vi "Begin.vi"(8 "error in":errorcluster) -> (0 "error out":errorcluster)   [LabVIEW 2020]
doc: "Called before other user functions, this VI is expected to open initial I/O refnums, load in file data, and do all program initialization. Notice that the <B>error out</B> terminal is simply used for data flow. Wiring it to other structures or subVIs ensures that this VI runs first."
uses:
  <vilib>/Rock Robotics/WPI/Compressor/WPI_CompressorFeedbackMode.ctl
  <vilib>/Rock Robotics/WPI/DriverStation/WPI_DriverStationRobotMode2.ctl
  <vilib>/Rock Robotics/WPI/Joystick/WPI_JoystickDeviceEnum.ctl
  <vilib>/Rock Robotics/WPI/ThirdParty/REV Robotics/REVLib/Typedef/Spark MAX Control Type.ctl
  <vilib>/Rock Robotics/WPI/ThirdParty/Sensors/navX/_TypeDefs/FRIC_navX_DeviceNumbersTypeDef.ctl
  <vilib>/Rock Robotics/WPI/Solenoid/WPI_SolenoidChannel.ctl
  <vilib>/Rock Robotics/SystemInterfaces/DIO/FPGA_DIOPWMChannel.ctl
  <vilib>/Rock Robotics/SystemInterfaces/DIO/FPGA_DIOChannel.ctl
  Robot Global Data.vi
  <vilib>/Rock Robotics/Network Tables/NT Write String Array.vi
  <vilib>/Rock Robotics/WPI/Solenoid/WPI_SolenoidOpenDouble.vi
  <vilib>/Rock Robotics/WPI/Utilities/WPI_GetSetVariantRefNum.vi
  <vilib>/Rock Robotics/WPI/MotorControl/WPI_MotorControlOpen SPARK.vi
  <vilib>/Rock Robotics/WPI/Switch/WPI_SwitchOpenLimit.vi
panel:
  in  "Feedback Configuration":T2={"Feedback Sensor"=enum."Analog Only", "Max Pressure (PSI)"=120.0, "Min Pressure (PSI)"=90.0}
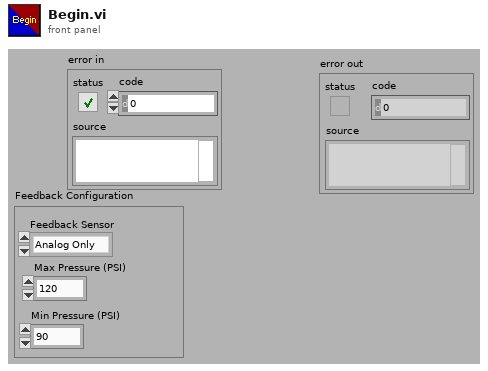
[diagram p1: front panel]
types:
  T1 = typedef "WPI_CompressorFeedbackMode.ctl" = enum16{"Analog Only", "Digital Only", "Hybrid"}
  T2 = cluster{"Feedback Sensor":T1, "Max Pressure (PSI)":dbl, "Min Pressure (PSI)":dbl}
  T3 = typedef "FPGA_DIOChannel.ctl" = enum8{"DIO 0", "DIO 1", "DIO 2", "DIO 3", "DIO 4", "DIO 5", "DIO 6", "DIO 7", "DIO 8", "DIO 9", "DIO MXP 0", "DIO MXP 1", "DIO MXP 2", "DIO MXP 3", "DIO MXP 4", "DIO MXP 5", "DIO MXP 6", "DIO MXP 7", "DIO MXP 8", "DIO MXP 9", "DIO MXP 10", "DIO MXP 11", "DIO MXP 12", "DIO MXP 13", "DIO MXP 14", "DIO MXP 15", "SPI Port CS1", "SPI Port CS2", "SPI Port CS3", "SPI Port MISO", "SPI Port MOSI", "Invalid"}
  T4 = typedef "FPGA_DIOPWMChannel.ctl" = enum8{"PWM 0", "PWM 1", "PWM 2", "PWM 3", "PWM 4", "PWM 5", "PWM 6", "PWM 7", "PWM 8", "PWM 9", "PWM MXP 0", "PWM MXP 1", "PWM MXP 2", "PWM MXP 3", "PWM MXP 4", "PWM MXP 5", "PWM MXP 6", "PWM MXP 7", "PWM MXP 8", "PWM MXP 9", "Invalid"}
  T5 = typedef "WPI_JoystickDeviceEnum.ctl" = enum16{"USB 0", "USB 1", "USB 2", "USB 3", "USB 4", "USB 5"}
  T6 = typedef "WPI_SolenoidChannel.ctl" = enum8{"Solenoid 0", "Solenoid 1", "Solenoid 2", "Solenoid 3", "Solenoid 4", "Solenoid 5", "Solenoid 6", "Solenoid 7", "Solenoid 8", "Solenoid 9", "Solenoid 10", "Solenoid 11", "Solenoid 12", "Solenoid 13", "Solenoid 14", "Solenoid 15", "Invalid"}
  T7 = typedef "Spark MAX Control Type.ctl" = enum16{"Percent VBus", "Voltage", "Velocity", "Position", "Smart Motion", "Current", "Smart Velocity"}
  T8 = typedef "FRIC_navX_DeviceNumbersTypeDef.ctl" = enum16{"Dev0", "Dev1", "Dev2", "Dev3"}
  T9 = typedef "WPI_DriverStationRobotMode2.ctl" = enum16{"Autonomous Disabled", "Autonomous Enabled", "Teleop Disabled", "Teleop Enabled", "Disconnected", "Finish", "Test Disabled", "Test Enabled", "Emergency Stopped"}
  T10 = typedef "WPI_SwitchDevRef.ctl" = cluster{"DevStatus":errorcluster, "DIO Channel":T3, "CntIndex":T11, "Normally Closed":bool}
  T11 = typedef "FPGA_CounterCtrSystemIndex.ctl" = enum8{"Ctr 0", "Ctr 1", "Ctr 2", "Ctr 3", "Ctr 4", "Ctr 5", "Ctr 6", "Ctr 7", "Invalid"}
  T12 = typedef "WPI_SolenoidDevRef.ctl" = cluster{"DevStatus":errorcluster, "Pneumatics Control Module":u8, "Forward Solenoid Channel":T6, "Reverse Solenoid Channel":T6}
  T13 = typedef "WPI_CompressorDevRef.ctl" = cluster{"DevStatus":errorcluster, "Pneumatics Control Module":u8}
  T14 = typedef "WPI_JoystickDevRef.ctl" = cluster{"Device":T5}
  T15 = typedef "WPI_MotorControlDeviceRef.ctl" = cluster{"DeviceStatus":errorcluster, "Type":T16, "PWM":cluster{"PWM Channel":T4, "DeadBand":T17}, "CAN":cluster{"Device Number":u8, "SetOutput VI Ref":variant, "GetOutput VI Ref":variant, "Enable VI Ref":variant, "Disable VI Ref":variant, "Data":variant}, "Invert":bool, "DIO PWM":cluster{"PWM \"Enable\" Channel":T4, "DIOChannel":T3, "PWM Rate":dbl}}
  T16 = typedef "WPI_MotorControlType.ctl" = enum16{"PWM", "CAN", "DIO PWM"}
  T17 = typedef "WPI_PWMDeadband.ctl" = cluster{"Name":string, "maxPositivePwm":i32, "minPositivePwm":i32, "centerPwm":i32, "maxNegativePwm":i32, "minNegativePwm":i32, "angularRange":u16}
  T18 = typedef "CTRE_Phoenix_CANcoder_DeviceRef.ctl" = cluster{"DeviceStatus":errorcluster, "Device Number":u8, "Handle":u64, "UsageFrame":u32, "Library Path":path}
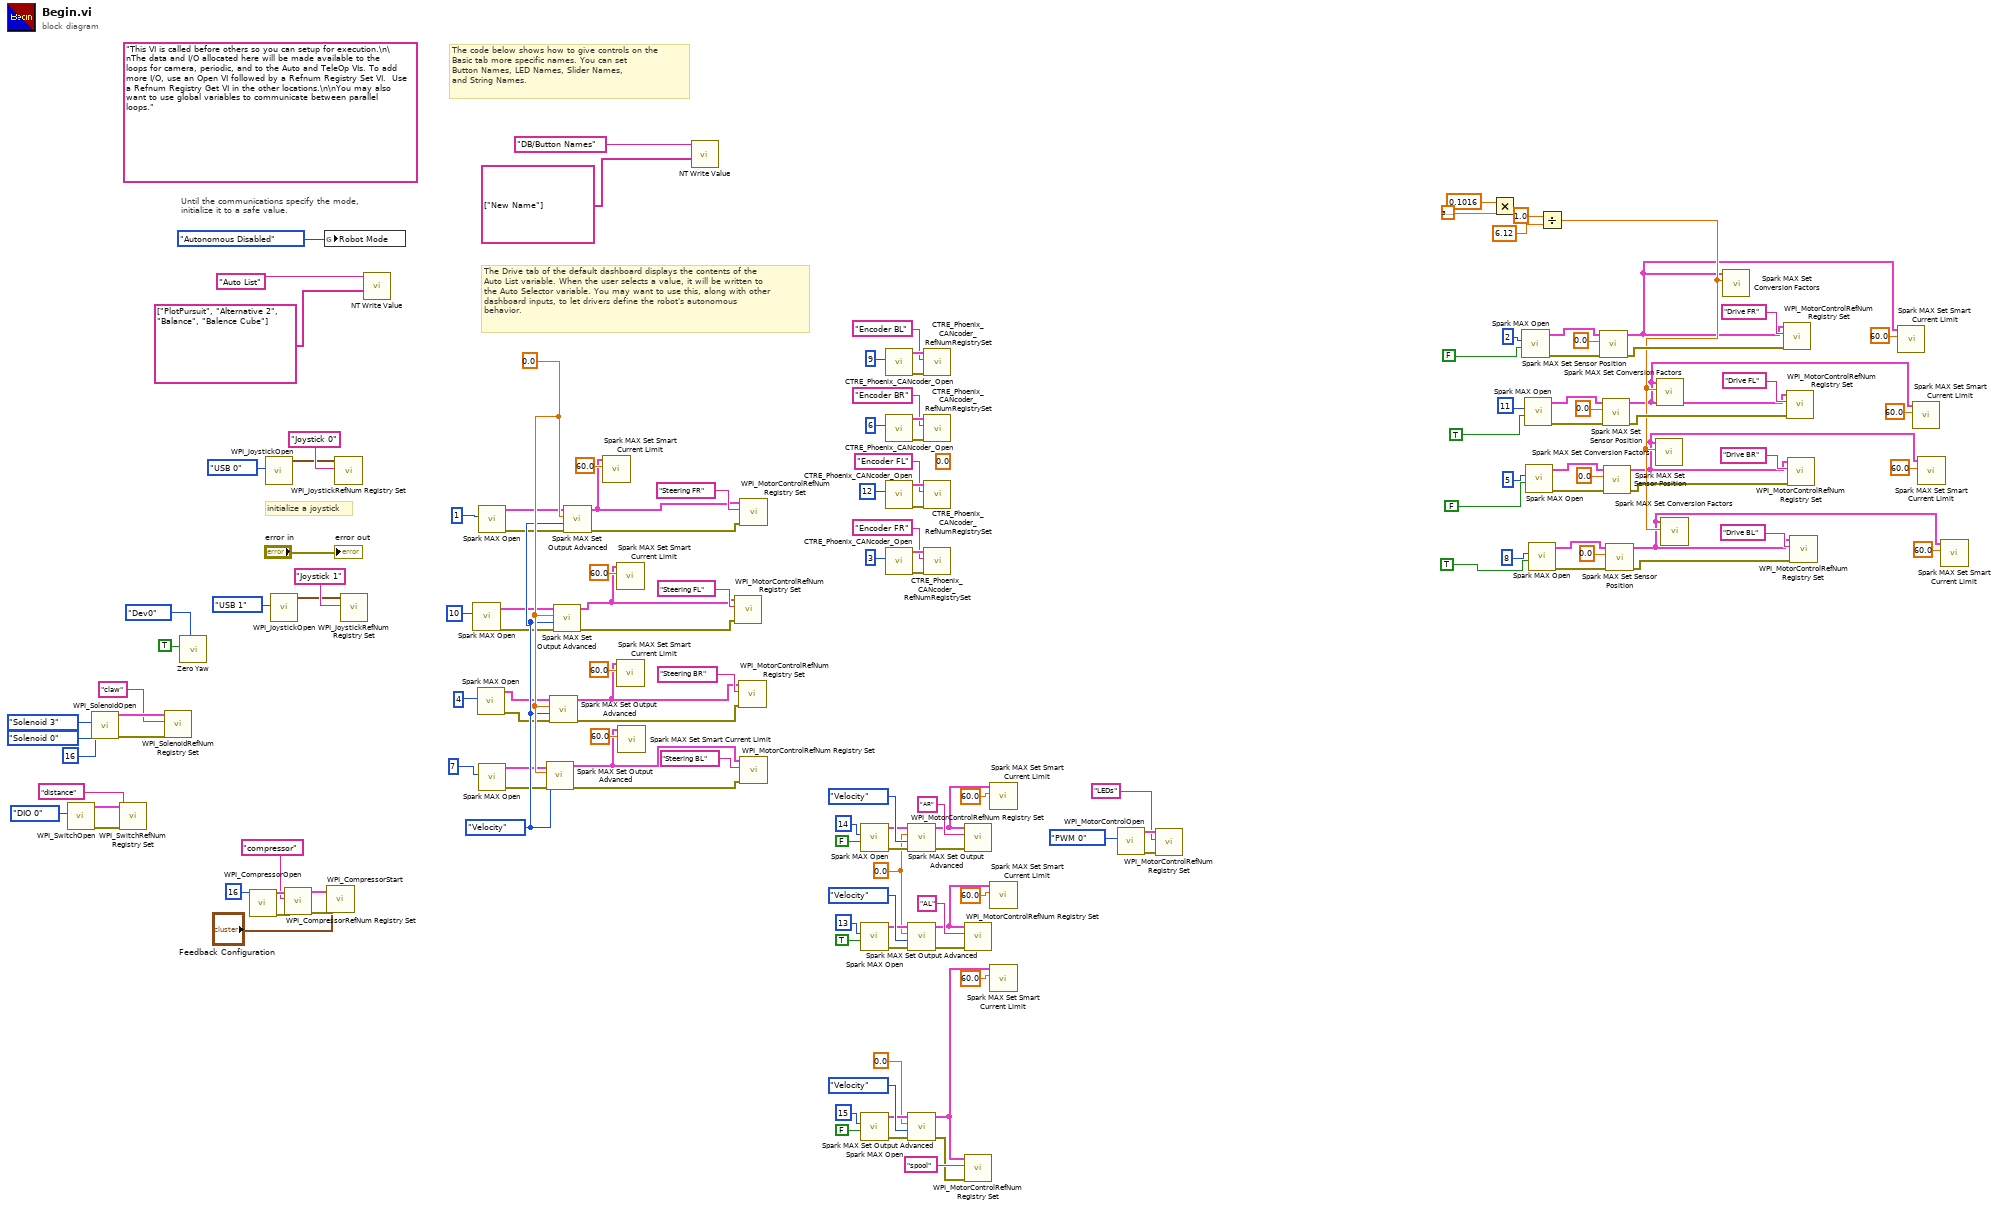
[diagram p0: block diagram]
diagram:
  w36 = 0.0 ("Setpoint")
  w93 = Spark_MAX_Control_Type."Velocity" ("Control Mode")
  (unwired) 0.0 ("Position")
  w94 = 0.0 ("New Position")
  (unwired) "This VI is called before others so you can setup for execution.\n\nThe data and I/O allocated here will be made available to the loops for camera, periodic, and to the Auto and TeleOp VIs. To add more I/O, use an Open VI followed by a Refnum Registry Set VI.  Use a Refnum Registry Get VI in the other locations.\n\nYou may also want to use global variables to communicate between parallel loops."
  # "The Drive tab of the default dashboard displays the contents of the\nAuto List variable. When the user selects a value, it will be written to\nthe Auto Selector variable. You may want to use this, along with other\ndashboard inputs, to let drivers define the robot's autonomous\nbehavior."
  # "The code below shows how to give controls on the\nBasic tab more specific names. You can set\nButton Names, LED Names, Slider Names,\nand String Names."
  # "initialize a joystick"
  # "Until the communications specify the mode,\ninitialize it to a safe value."
  n1 = call-poly <vilib>:"WPI_SwitchOpen.vi"("DIO Channel"=FPGA_DIOChannel."DIO 0") -> ("error out"=w3:errorcluster, "SwitchDevRef"=w2:T10)  [unwired: 9 in]
  n2 = call-poly <vilib>:"WPI_SolenoidOpen.vi"("Reverse Solenoid Channel"=WPI_SolenoidChannel."Solenoid 0", "Forward Solenoid Channel"=WPI_SolenoidChannel."Solenoid 3", "Pneumatics Device (def)"=u8 16) -> ("error out"=w20:errorcluster, "SolenoidDevRef"=w21:T12)  [unwired: 7 in]
  n3 = call <vilib>:"WPI_SwitchRefNum Registry Set.vi"("error in (no error)"=w3, "refnum name"="distance", "SwitchDevRef"=w2) -> ()  [unwired: 7 in, 2 out]
  n4 = call <vilib>:"WPI_SolenoidRefNum Registry Set.vi"("error in (no error)"=w20, "refnum name"="claw", "SolenoidDevRef"=w21) -> ()  [unwired: 7 in, 2 out]
  n5 = call <vilib>:"Zero Yaw.vi"("Device Number"=FRIC_navX_DeviceNumbersTypeDef."Dev0", "Zero"=TRUE) -> ()  [unwired: 10 in]
  n6 = call <vilib>:"WPI_CompressorOpen.vi"("Pneumatics device (def)"=u8 16) -> ("CompressorDevRef"=w25:T13, "error out"=w26:errorcluster)  [unwired: 13 in]
  n7 = call <vilib>:"WPI_JoystickOpen.vi"("JoystickDevice"=WPI_JoystickDeviceEnum."USB 0") -> ("JoystickDevRef"=w149:T14)  [unwired: 10 in]
  n8 = call <vilib>:"WPI_JoystickOpen.vi"("JoystickDevice"=WPI_JoystickDeviceEnum."USB 1") -> ("JoystickDevRef"=w10:T14)  [unwired: 10 in]
  n9 = call <vilib>:"WPI_CompressorRefNum Registry Set.vi"("error in (no error)"=w26, "refnum name"="compressor", "CompressorDevRef"=w25) -> ("error out"=w16:errorcluster, "CompressorDevRef"=w15:T13)  [unwired: 7 in]
  n10 = global write "Robot Global Data.vi" "Robot Mode"(WPI_DriverStationRobotMode2."Autonomous Disabled" ("Robot Mode")) -> ()
  n11 = call <vilib>:"WPI_CompressorStart.vi"("error in (no error)"=w16, "Feedback Configuration"="Feedback Configuration", "CompressorDevRef"=w15) -> ()  [unwired: 7 in, 2 out]
  n12 = call <vilib>:"WPI_JoystickRefNum Registry Set.vi"("refnum name"="Joystick 0", "JoystickDevRef"=w149) -> ()  [unwired: 8 in, 2 out]
  n13 = call <vilib>:"WPI_JoystickRefNum Registry Set.vi"("refnum name"="Joystick 1", "JoystickDevRef"=w10) -> ()  [unwired: 8 in, 2 out]
  n14 = call-poly <vilib>:"NT Write Value.vi"("value"=string[] ["PlotPursuit", "Alternative 2", "Balance", "Balence Cube"] ("String Array"), "name"="Auto List" ("Name")) -> ()  [unwired: 9 in, 1 out]
  n15 = call <vilib>:"Spark MAX Open.vi"("Device Number"=u8 10) -> ("error out"=w89:errorcluster, "MotorControlDeviceRef"=w90:T15)  [unwired: 9 in]
  n16 = call <vilib>:"Spark MAX Open.vi"("Device Number"=u8 4) -> ("error out"=w87:errorcluster, "MotorControlDeviceRef"=w88:T15)  [unwired: 9 in]
  n17 = call <vilib>:"Spark MAX Open.vi"("Device Number"=u8 1) -> ("error out"=w91:errorcluster, "MotorControlDeviceRef"=w92:T15)  [unwired: 9 in]
  n18 = call <vilib>:"Spark MAX Open.vi"("Device Number"=u8 7) -> ("error out"=w85:errorcluster, "MotorControlDeviceRef"=w86:T15)  [unwired: 9 in]
  n19 = call <vilib>:"Spark MAX Set Output Advanced.vi"("error in (no error)"=w85, "Control Mode"=w93, "Setpoint"=w94, "MotorControlDevRef"=w86) -> ("error out"=w84:errorcluster, "MotorControlDevRef"=w54:T15)  [unwired: 6 in]
  n20 = call <vilib>:"Spark MAX Set Output Advanced.vi"("error in (no error)"=w87, "Control Mode"=w93, "Setpoint"=w94, "MotorControlDevRef"=w88) -> ("error out"=w83:errorcluster, "MotorControlDevRef"=w55:T15)  [unwired: 6 in]
  n21 = call <vilib>:"Spark MAX Set Output Advanced.vi"("error in (no error)"=w89, "Control Mode"=w93, "Setpoint"=w94, "MotorControlDevRef"=w90) -> ("error out"=w82:errorcluster, "MotorControlDevRef"=w57:T15)  [unwired: 6 in]
  n22 = call <vilib>:"Spark MAX Set Output Advanced.vi"("error in (no error)"=w91, "Control Mode"=w93, "Setpoint"=w94, "MotorControlDevRef"=w92) -> ("error out"=w81:errorcluster, "MotorControlDevRef"=w56:T15)  [unwired: 6 in]
  n23 = call <vilib>:"Spark MAX Set Smart Current Limit.vi"("Primay Current Limit (80A)"=60.0, "MotorControlDeviceRef in"=w56) -> ()  [unwired: 8 in, 2 out]
  n24 = call <vilib>:"Spark MAX Set Smart Current Limit.vi"("Primay Current Limit (80A)"=60.0, "MotorControlDeviceRef in"=w57) -> ()  [unwired: 8 in, 2 out]
  n25 = call <vilib>:"Spark MAX Set Smart Current Limit.vi"("Primay Current Limit (80A)"=60.0, "MotorControlDeviceRef in"=w55) -> ()  [unwired: 8 in, 2 out]
  n26 = call <vilib>:"Spark MAX Set Smart Current Limit.vi"("Primay Current Limit (80A)"=60.0, "MotorControlDeviceRef in"=w54) -> ()  [unwired: 8 in, 2 out]
  n27 = call-poly <vilib>:"NT Write Value.vi"("value"=string[] ["New Name"], "name"="DB/Button Names" ("Name")) -> ()  [unwired: 9 in, 1 out]
  n28 = call <vilib>:"WPI_MotorControlRefNum Registry Set.vi"("error in (no error)"=w82, "refnum name"="Steering FL", "MotorControlDevRef"=w57) -> ()  [unwired: 7 in, 2 out]
  n29 = call <vilib>:"WPI_MotorControlRefNum Registry Set.vi"("error in (no error)"=w83, "refnum name"="Steering BR", "MotorControlDevRef"=w55) -> ()  [unwired: 7 in, 2 out]
  n30 = call <vilib>:"WPI_MotorControlRefNum Registry Set.vi"("error in (no error)"=w81, "refnum name"="Steering FR", "MotorControlDevRef"=w56) -> ()  [unwired: 7 in, 2 out]
  n31 = call <vilib>:"WPI_MotorControlRefNum Registry Set.vi"("error in (no error)"=w84, "refnum name"="Steering BL", "MotorControlDevRef"=w54) -> ()  [unwired: 7 in, 2 out]
  n32 = call <vilib>:"Spark MAX Open.vi"("Invert"=FALSE, "Device Number"=u8 14) -> ("error out"=w43:errorcluster, "MotorControlDeviceRef"=w44:T15)  [unwired: 8 in]
  n33 = call <vilib>:"Spark MAX Open.vi"("Invert"=TRUE, "Device Number"=u8 13) -> ("error out"=w49:errorcluster, "MotorControlDeviceRef"=w50:T15)  [unwired: 8 in]
  n34 = call <vilib>:"Spark MAX Open.vi"("Invert"=FALSE, "Device Number"=u8 15) -> ("error out"=w30:errorcluster, "MotorControlDeviceRef"=w31:T15)  [unwired: 8 in]
  n35 = call <vilib>:"CTRE_Phoenix_CANcoder_Open.vi"("Device Number"=u8 9) -> ("error out"=w130:errorcluster, "CTRE_CANcoder_DeviceRef"=w129:T18)  [unwired: 9 in]
  n36 = call <vilib>:"CTRE_Phoenix_CANcoder_Open.vi"("Device Number"=u8 6) -> ("error out"=w134:errorcluster, "CTRE_CANcoder_DeviceRef"=w133:T18)  [unwired: 9 in]
  n37 = call <vilib>:"CTRE_Phoenix_CANcoder_Open.vi"("Device Number"=u8 12) -> ("error out"=w138:errorcluster, "CTRE_CANcoder_DeviceRef"=w137:T18)  [unwired: 9 in]
  n38 = call <vilib>:"CTRE_Phoenix_CANcoder_Open.vi"("Device Number"=u8 3) -> ("error out"=w142:errorcluster, "CTRE_CANcoder_DeviceRef"=w141:T18)  [unwired: 9 in]
  n39 = call <vilib>:"Spark MAX Set Output Advanced.vi"("error in (no error)"=w43, "Control Mode"=Spark_MAX_Control_Type."Velocity", "Setpoint"=w36, "MotorControlDevRef"=w44) -> ("error out"=w42:errorcluster, "MotorControlDevRef"=w41:T15)  [unwired: 6 in]
  n40 = call <vilib>:"Spark MAX Set Output Advanced.vi"("error in (no error)"=w49, "Control Mode"=Spark_MAX_Control_Type."Velocity", "Setpoint"=w36, "MotorControlDevRef"=w50) -> ("error out"=w48:errorcluster, "MotorControlDevRef"=w40:T15)  [unwired: 6 in]
  n41 = call <vilib>:"Spark MAX Set Output Advanced.vi"("error in (no error)"=w30, "Control Mode"=Spark_MAX_Control_Type."Velocity", "Setpoint"=0.0, "MotorControlDevRef"=w31) -> ("error out"=w12:errorcluster, "MotorControlDevRef"=w13:T15)  [unwired: 6 in]
  n42 = call <vilib>:"CTRE_Phoenix_CANcoder_RefNumRegistrySet.vi"("error in (no error)"=w130, "refnum name"="Encoder BL", "CTRE_CANcoder_DeviceRef"=w129) -> ()  [unwired: 7 in, 2 out]
  n43 = call <vilib>:"CTRE_Phoenix_CANcoder_RefNumRegistrySet.vi"("error in (no error)"=w134, "refnum name"="Encoder BR", "CTRE_CANcoder_DeviceRef"=w133) -> ()  [unwired: 7 in, 2 out]
  n44 = call <vilib>:"CTRE_Phoenix_CANcoder_RefNumRegistrySet.vi"("error in (no error)"=w138, "refnum name"="Encoder FL", "CTRE_CANcoder_DeviceRef"=w137) -> ()  [unwired: 7 in, 2 out]
  n45 = call <vilib>:"CTRE_Phoenix_CANcoder_RefNumRegistrySet.vi"("error in (no error)"=w142, "refnum name"="Encoder FR", "CTRE_CANcoder_DeviceRef"=w141) -> ()  [unwired: 7 in, 2 out]
  n46 = call <vilib>:"WPI_MotorControlRefNum Registry Set.vi"("error in (no error)"=w42, "refnum name"="AR", "MotorControlDevRef"=w41) -> ()  [unwired: 7 in, 2 out]
  n47 = call <vilib>:"WPI_MotorControlRefNum Registry Set.vi"("error in (no error)"=w48, "refnum name"="AL", "MotorControlDevRef"=w40) -> ()  [unwired: 7 in, 2 out]
  n48 = call <vilib>:"WPI_MotorControlRefNum Registry Set.vi"("error in (no error)"=w12, "refnum name"="spool", "MotorControlDevRef"=w13) -> ()  [unwired: 7 in, 2 out]
  n49 = call <vilib>:"Spark MAX Set Smart Current Limit.vi"("Primay Current Limit (80A)"=60.0, "MotorControlDeviceRef in"=w41) -> ()  [unwired: 8 in, 2 out]
  n50 = call <vilib>:"Spark MAX Set Smart Current Limit.vi"("Primay Current Limit (80A)"=60.0, "MotorControlDeviceRef in"=w40) -> ()  [unwired: 8 in, 2 out]
  n51 = call <vilib>:"Spark MAX Set Smart Current Limit.vi"("Primay Current Limit (80A)"=60.0, "MotorControlDeviceRef in"=w13) -> ()  [unwired: 8 in, 2 out]
  n52 = call-poly <vilib>:"WPI_MotorControlOpen.vi"("PWM Channel"=FPGA_DIOPWMChannel."PWM 0") -> ("error out"=w7:errorcluster, "MotorControlDeviceRef"=w6:T15)  [unwired: 9 in]
  n53 = call <vilib>:"WPI_MotorControlRefNum Registry Set.vi"("error in (no error)"=w7, "refnum name"="LEDs", "MotorControlDevRef"=w6) -> ()  [unwired: 7 in, 2 out]
  n54 = Multiply(x=0.1016, y=3.141592653589793) -> ()  [unwired: 1 out]
  n55 = call <vilib>:"Spark MAX Open.vi"("Invert"=FALSE, "Device Number"=u8 2) -> ("error out"=w116:errorcluster, "MotorControlDeviceRef"=w117:T15)  [unwired: 8 in]
  n56 = call <vilib>:"Spark MAX Open.vi"("Invert"=TRUE, "Device Number"=u8 11) -> ("error out"=w112:errorcluster, "MotorControlDeviceRef"=w113:T15)  [unwired: 8 in]
  n57 = call <vilib>:"Spark MAX Open.vi"("Invert"=FALSE, "Device Number"=u8 5) -> ("error out"=w108:errorcluster, "MotorControlDeviceRef"=w109:T15)  [unwired: 8 in]
  n58 = call <vilib>:"Spark MAX Open.vi"("Invert"=TRUE, "Device Number"=u8 8) -> ("error out"=w104:errorcluster, "MotorControlDeviceRef"=w105:T15)  [unwired: 8 in]
  n59 = Divide(x=1.0, y=6.12) -> (x/y=w70:dbl)
  n60 = call <vilib>:"Spark MAX Set Sensor Position.vi"("error in"=w116, "Position"=0.0 ("New Position"), "MotorControlDeviceRef"=w117) -> ("error out"=w115:errorcluster, "MotorControlDeviceRef"=w61:T15)  [unwired: 7 in]
  n61 = call <vilib>:"Spark MAX Set Sensor Position.vi"("error in"=w112, "Position"=0.0 ("New Position"), "MotorControlDeviceRef"=w113) -> ("error out"=w111:errorcluster, "MotorControlDeviceRef"=w60:T15)  [unwired: 7 in]
  n62 = call <vilib>:"Spark MAX Set Sensor Position.vi"("error in"=w108, "Position"=0.0 ("New Position"), "MotorControlDeviceRef"=w109) -> ("error out"=w107:errorcluster, "MotorControlDeviceRef"=w59:T15)  [unwired: 7 in]
  n63 = call <vilib>:"Spark MAX Set Sensor Position.vi"("error in"=w104, "Position"=0.0 ("New Position"), "MotorControlDeviceRef"=w105) -> ("error out"=w103:errorcluster, "MotorControlDeviceRef"=w58:T15)  [unwired: 7 in]
  n64 = call <vilib>:"Spark MAX Set Conversion Factors.vi"("Position Factor (1)"=w70, "MotorControlDeviceRef in"=w59) -> ()  [unwired: 8 in, 2 out]
  n65 = call <vilib>:"Spark MAX Set Conversion Factors.vi"("Position Factor (1)"=w70, "MotorControlDeviceRef in"=w60) -> ()  [unwired: 8 in, 2 out]
  n66 = call <vilib>:"Spark MAX Set Conversion Factors.vi"("Position Factor (1)"=w70, "MotorControlDeviceRef in"=w58) -> ()  [unwired: 8 in, 2 out]
  n67 = call <vilib>:"Spark MAX Set Conversion Factors.vi"("Position Factor (1)"=w70, "MotorControlDeviceRef in"=w61) -> ()  [unwired: 8 in, 2 out]
  n68 = call <vilib>:"WPI_MotorControlRefNum Registry Set.vi"("error in (no error)"=w115, "refnum name"="Drive FR", "MotorControlDevRef"=w61) -> ()  [unwired: 7 in, 2 out]
  n69 = call <vilib>:"WPI_MotorControlRefNum Registry Set.vi"("error in (no error)"=w111, "refnum name"="Drive FL", "MotorControlDevRef"=w60) -> ()  [unwired: 7 in, 2 out]
  n70 = call <vilib>:"WPI_MotorControlRefNum Registry Set.vi"("error in (no error)"=w107, "refnum name"="Drive BR", "MotorControlDevRef"=w59) -> ()  [unwired: 7 in, 2 out]
  n71 = call <vilib>:"WPI_MotorControlRefNum Registry Set.vi"("error in (no error)"=w103, "refnum name"="Drive BL", "MotorControlDevRef"=w58) -> ()  [unwired: 7 in, 2 out]
  n72 = call <vilib>:"Spark MAX Set Smart Current Limit.vi"("Primay Current Limit (80A)"=60.0, "MotorControlDeviceRef in"=w61) -> ()  [unwired: 8 in, 2 out]
  n73 = call <vilib>:"Spark MAX Set Smart Current Limit.vi"("Primay Current Limit (80A)"=60.0, "MotorControlDeviceRef in"=w60) -> ()  [unwired: 8 in, 2 out]
  n74 = call <vilib>:"Spark MAX Set Smart Current Limit.vi"("Primay Current Limit (80A)"=60.0, "MotorControlDeviceRef in"=w59) -> ()  [unwired: 8 in, 2 out]
  n75 = call <vilib>:"Spark MAX Set Smart Current Limit.vi"("Primay Current Limit (80A)"=60.0, "MotorControlDeviceRef in"=w58) -> ()  [unwired: 8 in, 2 out]
  "error out" <- "error in"
